vi "UDP&Screen.vi"() -> ()   [LabVIEW 2021]
uses:
  <resource>/objmgr/IMAQImage.rc
  <vilib>/vision/Image Controls.llb/IMAQ Image.ctl
panel:
  out "Image Type":u32(ring) items=["Grayscale (U8)", "Grayscale (I16)", "Grayscale (SGL)", "Complex (CSG)", "RGB (U32)", "HSL (U32)", "RGB (U64)", "Grayscale (U16)"]
  out "Image Size 2":cluster{"x":i32, "y":i32}
  out "Image":T1
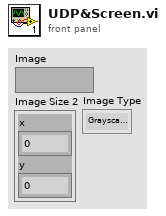
[diagram p1: front panel]
types:
  T1 = typedef "IMAQ Image.ctl" = refnum<image>
  T2 = typedef "Image Type" = u32
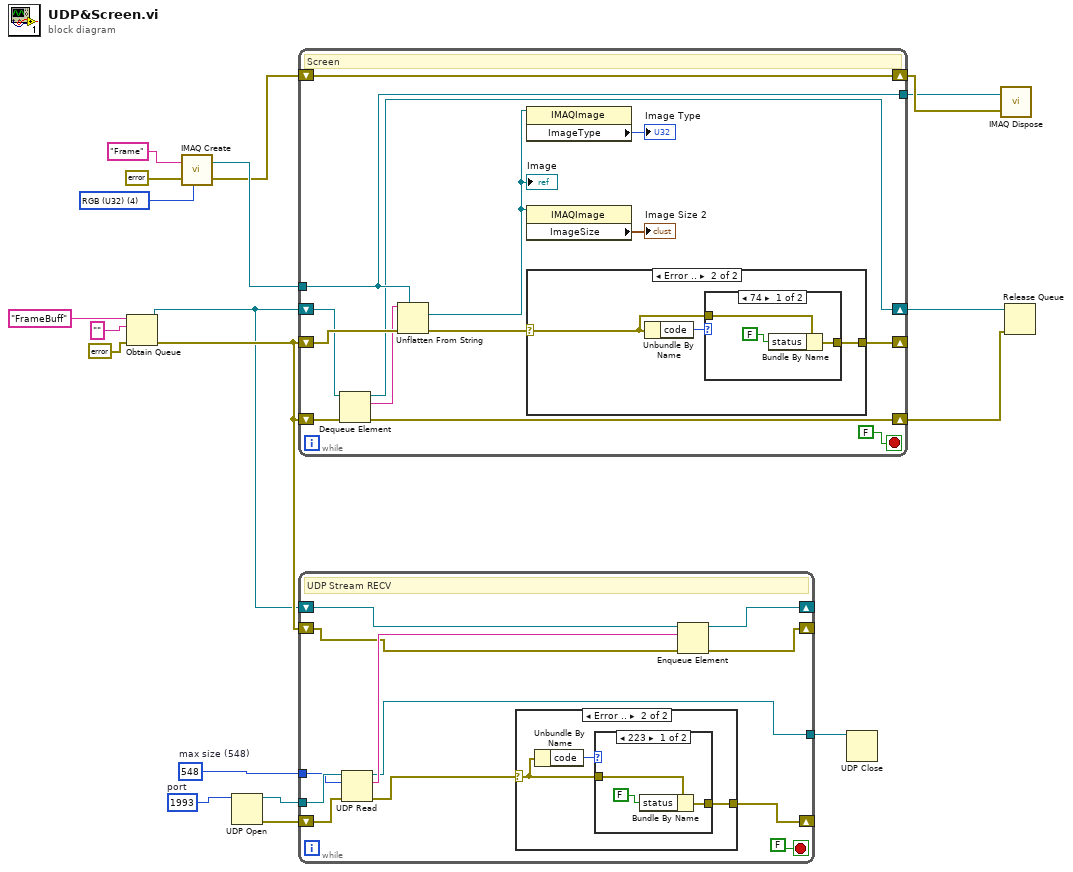
[diagram p0: block diagram]
diagram:
  w5 = 548  # max size (548)
  w8 = u16 1993  # port
  w17 = T2 4 items=["Grayscale (U8)", "Grayscale (I16)", "Grayscale (SGL)", "Complex (CSG)", "RGB (U32)", "HSL (U32)", "RGB (U64)", "Grayscale (U16)"] ("Image Type")
  n1 = Obtain Queue(name (unnamed)="FrameBuff", element data type="", error in (no error)=errorcluster {"status"=FALSE, "code"=0, "source"=""}) -> (queue out=w2:refnum<queue>, error out=w4:errorcluster)  [unwired: 2 in, 1 out]
  n2 = call "IMAQ Create"("Image Name"="Frame", "Image Type"=w17, "error in (no error)"=errorcluster {"status"=FALSE, "code"=0, "source"=""}) -> ("New Image"=w14:T1, "error out"=w3:errorcluster)  [unwired: 2 in]
  n3 = UDP Open(11:w8) -> (port=w6:refnum<k16>, 0:w7:errorcluster)  [unwired: 4 in, 1 out]
  n4 = while {
    shift-right: [w30] -> w13
    shift-left: w3 -> [w30]
    shift-right: [w28] -> w11
    shift-left: w4 -> [w32]
    shift-right: [w27] -> w10
    shift-left: w2 -> [w31]
    shift-right: [w25] -> _
    shift-left: w4 -> [w33]
    tunnel: w14 -> [w29]
    tunnel: [w29] -> w12
    stop <- FALSE stop-if-true
    # "Screen"
    n5 = Dequeue Element(queue=w31, error in (no error)=w32) -> (queue out=w27:refnum<queue>, element=w21:string, error out=w28:errorcluster)  [unwired: 1 in, 1 out]
    n6 = Unflatten From String(type=w29, binary string=w21, error in (no error)=w33) -> (value=w24:T1, error out=w26:errorcluster)  [unwired: 2 in, 1 out]
    "Image" <- w24
    n7 = property class="IMAQImage"(reference=w24) -> ("ImageType"=→"Image Type":u32)  [unwired: 1 in, 2 out]
    n8 = property class="IMAQImage"(reference=w24) -> ("ImageSize"=→"Image Size 2":cluster{"x":i32, "y":i32})  [unwired: 1 in, 2 out]
    n9 = case shown="Error .." w26 {
      selector: w26 -> [_ w34]
      tunnel: [_ w36] -> w25
      frame No Error {
      }
      frame Error {
        n10 = Unbundle By Name(w34) -> ("code"=w35:i32)
        n11 = case shown="74" w35 {
          tunnel: [w38 _] -> w36
          tunnel: w34 -> [w37 _]
          frame 74 {
            n12 = Bundle By Name(cluster=w37, "status"=FALSE) -> (w38:errorcluster)
          }
          frame 1 {
          }
        }
      }
    }
  }
  n13 = while {
    shift-right: [w47] -> _
    shift-left: w7 -> [w51]
    tunnel: w6 -> [w50]
    tunnel: w5 -> [w49]
    shift-right: [w45] -> _
    shift-left: w4 -> [w42]
    shift-right: [w46] -> _
    shift-left: w2 -> [w43]
    tunnel: [w41] -> w1
    stop <- FALSE stop-if-true
    # "UDP Stream RECV"
    n14 = UDP Read(connection ID=w50, max size (548)=w49, 8:w51) -> (data out=w44:string, error out=w48:errorcluster, 3:w41:refnum<k16>)  [unwired: 1 in, 2 out]
    n15 = case shown="Error .." w48 {
      selector: w48 -> [_ w52]
      tunnel: [_ w54] -> w47
      frame No Error {
      }
      frame Error {
        n16 = Unbundle By Name(w52) -> ("code"=w53:i32)
        n17 = case shown="223" w53 {
          tunnel: [w56 _] -> w54
          tunnel: w52 -> [w55 _]
          frame 223 {
            n18 = Bundle By Name(cluster=w55, "status"=FALSE) -> (w56:errorcluster)
          }
          frame 1 {
          }
        }
      }
    }
    n19 = Enqueue Element(queue=w43, element=w44, error in (no error)=w42) -> (queue out=w46:refnum<queue>, error out=w45:errorcluster)  [unwired: 1 in, 1 out]
  }
  n20 = UDP Close(connection ID=w1) -> ()  [unwired: 1 in, 2 out]
  n21 = call "IMAQ Dispose"("Image"=w12, "error in (no error)"=w13) -> ()  [unwired: 4 in, 1 out]
  n22 = Release Queue(queue=w10, error in (no error)=w11) -> ()  [unwired: 1 in, 3 out]
